vi "Actor Core.vi"(8 "error in":errorcluster, 11 "Test Actor in":refnum<class "Test Actor.lvclass">) -> (0 "error out":errorcluster, 3 "Actor out":refnum<class "Actor.lvclass">)   [LabVIEW 2020, in "Test.lvlib" / "Test Actor.lvclass"]
doc: "(<B>Filename</B>: Actor Framework.lvlib:Actor.lvclass:Actor Core.vi)\n\nReceives messages to the actor, reacts to them, and initiates any error handling that may shut the actor down.\n\nDescendant classes may override this VI to append parallel tasks for the actor to complete while it handles messages. Overrides use the Call Parent Method node."
uses:
  Test Actor.lvclass
  C:/Current projects/WS/PPL/HDH.Actor Framework.Core.Actor.lvlibp/1abvi3w/vi.lib/ActorFramework/Actor/Actor.lvclass
  PPL/HDH.Actor Framework.Core.Actor.lvlibp/1abvi3w/vi.lib/ActorFramework/Actor/Actor.lvclass
  PPL/HDH.Actor Framework.Core.Publisher.lvlibp/Messages/Response Msg/Response Core/Controls/Ctl_SendFunction.ctl
  PPL/HDH.Actor Framework.Core.Data Tracker.lvlibp/Messages for this Actor/Data Tracker Msg/Controls/Ctl_Action.ctl
  Test Actor.lvclass/Test Actor.ctl
  PPL/HDH.Actor Framework.Core.Graph.lvlibp/Graph/Graph.lvclass
  PPL/HDH.Actor Framework.Core.File Writer.lvlibp/File Writer/File Writer.lvclass
  PPL/HDH.Actor Framework.Core.File Writer.lvlibp/File Writer/File Post Action/File Post Action.lvclass
  Message/Test Instrument Msg/Test Instrument Msg.lvclass
  C:/Current projects/WS/PPL/HDH.Actor Framework.Core.Instrument Handler.lvlibp/Messages/Instrument Msg/Instrument Msg.lvclass
  Message/Test Multi Instrument Msg/Test Multi Instrument Msg.lvclass
  Message/Test Nested Multi Instrument Msg/Test Nested Multi Instrument Msg.lvclass
  PPL/HDH.Actor Framework.Core.Instrument Handler.lvlibp/Instrument Handler/Instrument Handler.lvclass
  PPL/HDH.Actor Framework.Core.Data Tracker.lvlibp/Data Tracker/Data Tracker.lvclass
  PPL/HDH.Actor Framework.Core.Actor.lvlibp/1abvi3w/vi.lib/ActorFramework/Message Enqueuer/Message Priority.ctl
  PPL/HDH.Actor Framework.Core.Data Tracker.lvlibp/Data Tracker/Data/Tracker Data.lvclass
  Message/Test Double Data Tracker/Test Double Data Tracker.lvclass
  C:/Current projects/WS/PPL/HDH.Actor Framework.Core.Publisher.lvlibp/Messages/Response Msg/Response Msg.lvclass
  Instrument/Test Instrument/Test Instrument.lvclass
  PPL/HDH.Actor Framework.Core.Instrument Driver.lvlibp/Instrument Driver/Controls/Ctl_ConnectionType.ctl
  Data/Test Double Data/Test Double Data.lvclass/Test Double Data.ctl
  Data/Test Double Data/Test Double Data.lvclass
  PPL/HDH.Actor Framework.Core.Msg.lvlibp/Sub Panel Insertion Msg/Sub Panel Insertion Msg.lvclass
  C:/Current projects/WS/PPL/HDH.Actor Framework.Core.Actor.lvlibp/1abvi3w/vi.lib/ActorFramework/Message/Message.lvclass
  PPL/HDH.Actor Framework.Core.File Writer.lvlibp/File Writer Messages/Open File Msg/Open File Msg.lvclass
  PPL/HDH.Actor Framework.Core.File Writer.lvlibp/File Writer Messages/Close File Msg/Close File Msg.lvclass
  PPL/HDH.Actor Framework.Core.Instrument Handler.lvlibp/Messages/Instrument Msg/Instrument Msg.lvclass
  PPL/HDH.Actor Framework.Core.Publisher.lvlibp/Publisher Messages/Targetted Msg/Targetted Msg.lvclass
  C:/Current projects/WS/PPL/HDH.Actor Framework.Core.Publisher.lvlibp/Publisher Messages/Sender Msg/Sender Msg.lvclass
  PPL/HDH.Actor Framework.Core.Instrument Handler.lvlibp/Instrument Handler Messages/Register Instrument Msg/Register Instrument Msg.lvclass
  PPL/HDH.Actor Framework.Core.Sequencer.lvlibp/Sequencer/Sequencer.lvclass
  PPL/HDH.Data.Generic.lvlibp/Data.lvclass
  PPL/HDH.Data.Generic.lvlibp/Generic Data/Generic Data.lvclass
  PPL/HDH.Actor Framework.Core.Actor.lvlibp/1abvi3w/vi.lib/ActorFramework/Stop Msg/Stop Msg.lvclass
  PPL/HDH.Actor Framework.Core.Sequencer.lvlibp
  PPL/HDH.Actor Framework.Core.Actor.lvlibp/1abvi3w/vi.lib/ActorFramework/Message Enqueuer/Message Enqueuer.lvclass
  PPL/HDH.Actor Framework.Core.Publisher.lvlibp/Publisher Messages/Publish Msg/Publish Msg.lvclass
  PPL/HDH.Actor Framework.Core.Instrument Driver.lvlibp/Instrument Driver/Instrument Driver.lvclass
  PPL/HDH.Actor Framework.Core.Publisher.lvlibp/Messages/Response Msg/Response Msg.lvclass
  PPL/HDH.Actor Framework.Core.Data Repository.lvlibp
  PPL/HDH.Actor Framework.Core.Data Tracker.lvlibp/Messages for this Actor/Data Tracker Msg/Data Tracker Msg.lvclass
  C:/Current projects/WS/PPL/HDH.Actor Framework.Core.Sequencer.lvlibp/Sequencer/Sequencer.lvclass
  C:/Current projects/WS/PPL/HDH.Actor Framework.Core.Data Tracker.lvlibp/Messages for this Actor/Data Tracker Msg/Data Tracker Msg.lvclass
  C:/Current projects/WS/PPL/HDH.Data.Generic.lvlibp/Data.lvclass
  PPL/HDH.Actor Framework.Core.Sequencer.lvlibp/Sequencer Messages/Batch Msg/Batch Msg.lvclass
  PPL/HDH.Actor Framework.Core.Publisher.lvlibp
  PPL/HDH.Actor Framework.Core.Data Tracker.lvlibp
panel:
  in  "Tab Control":T1(tab)
  in  "Send to tracker":bool
  in  "Send Function - Data Tracker":T2
  in  "Timeout if waiting(-1ms) - Data Tracker":i32=-1
  in  "Action(Start)":T3
  out "Data":string[](array[string])
  in  "Show data from repository":bool
  out "Success?":bool
  out "Found 'Test Double Data'":waveform(dbl)[](array[waveform])
  in  "Show data":bool
  in  "Stop Save":bool
  in  "Start Save":bool
  in  "File Path Control":path
  in  "Data":dbl[](array[numeric])
  in  "Publish Data to Graph":bool
  in  "Insert Graph":bool
  out "Recieved Data":waveform(dbl)[](graph)
  in  "Create Instrument":bool
  in  "Send Instrument Msg":bool
  in  "Publish Data?":bool=TRUE
  in  "Timeout if waiting(-1ms)":i32=-1
  in  "Send Function":T2
  in  "Msg Type":T4(ring)=enum."Test Nested Multi Instrument Msg"
  in  "Commit":bool
  in  "Setup Name":string
  in  "Single element?":bool
  in  "Tab Control 2":enum32{"String", "Double"}(tab)
  in  "String Array":string[](array[string])
  in  "Double Array":dbl[](array[numeric])
  out "replaced?":bool
  in  "Play Sequence":bool
  in  "Stop":bool
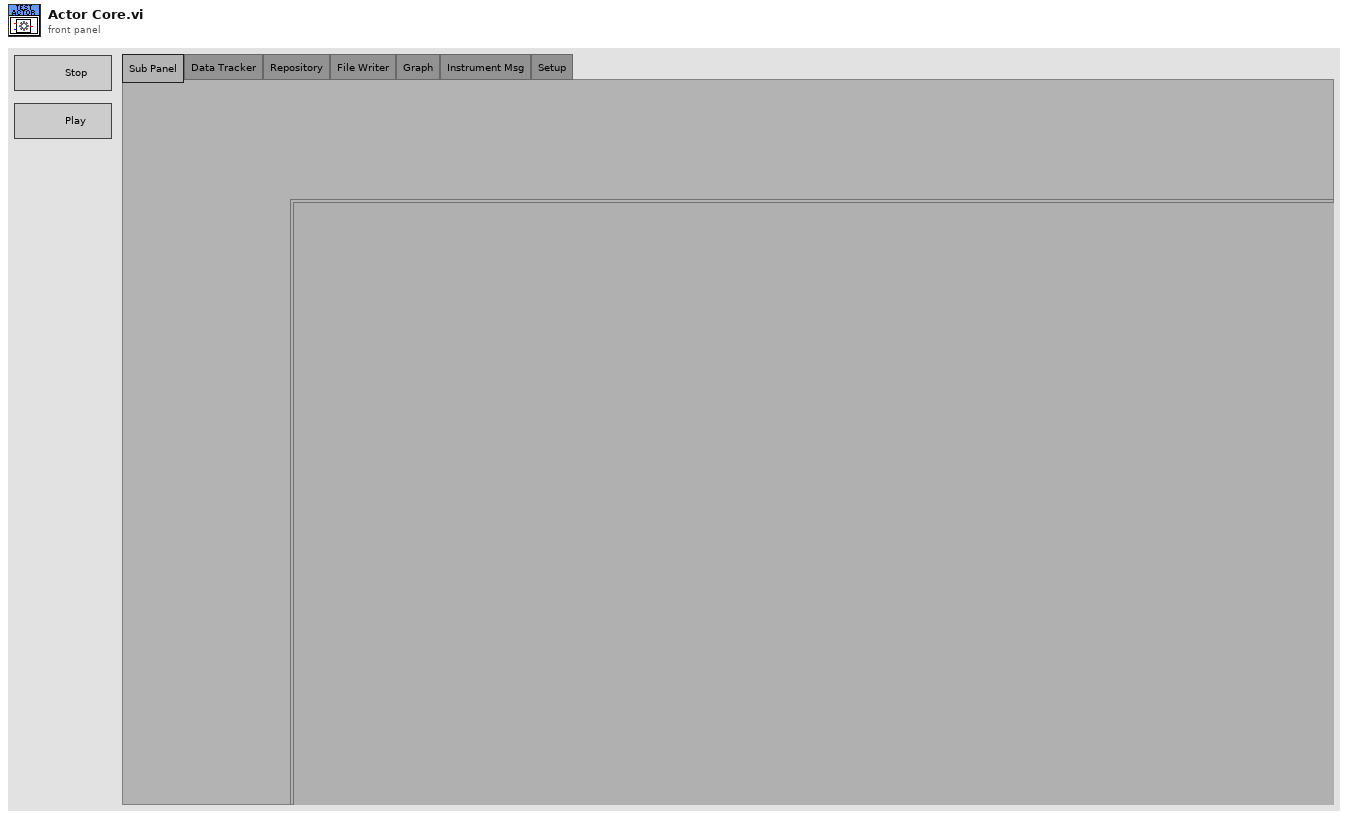
[diagram p1: front panel]
types:
  T1 = enum32{"Sub Panel", "Data Tracker", "Repository", "File Writer", "Graph", "Instrument Msg", "Setup"}
  T2 = typedef "HDH.Actor Framework.Core.Publisher.lvlibp/Ctl_SendFunction.ctl" = enum16{"Send and Forget", "Request Reply", "Await Reply"}
  T3 = typedef "HDH.Actor Framework.Core.Data Tracker.lvlibp/Ctl_Action.ctl" = enum16{"Start Tracking", "End Tracking", "Abort Tracking"}
  T4 = enum16{"Test Instrument Msg", "Test Multi Instrument Msg", "Test Nested Multi Instrument Msg"}
  T5 = enum32{"Invalid", "Standard", "Closed", "Hidden", "Minimized", "Maximized"}
  T6 = typedef "HDH.Actor Framework.Core.Instrument Driver.lvlibp/Instrument Driver.lvclass/Ctl_ConnectionType.ctl" = enum16{"BuiltIn/System", "PXI/PCI", "USB", "GPIB", "VXI", "Serial", "TCP/IP", "cRIO", "SCXI", "cDAQ", "SwitchBlock", "SCC", "FireWire", "Accessory", "CAN", "SwitchBlock Device"}
  T7 = typedef "HDH.Actor Framework.Core.Actor.lvlibp/Message Enqueuer.lvclass/Message Priority.ctl" = enum16{"Low", "Normal", "High"}
  T8 = typedef "HDH.Actor Framework.Core.Sequencer.lvlibp/Ctl_SequenceElement.ctl" = cluster{"Message Base Name":string, "Message Path":path, "Supports Data Access?":bool, "List Symbol":i32, "Sequence Control Element Array":T9[]}
  T9 = typedef "HDH.Actor Framework.Core.Sequencer.lvlibp/Ctl_SequenceControlElement.ctl" = cluster{"Data Override name":string, "Looped Override?":bool, "Control element":T10, "List Symbol":i32}
  T10 = typedef "HDH.Actor Framework.Core.Msg.lvlibp/Ctl_Control Element.ctl" = cluster{"Index":i32, "Label":string, "Value":variant}
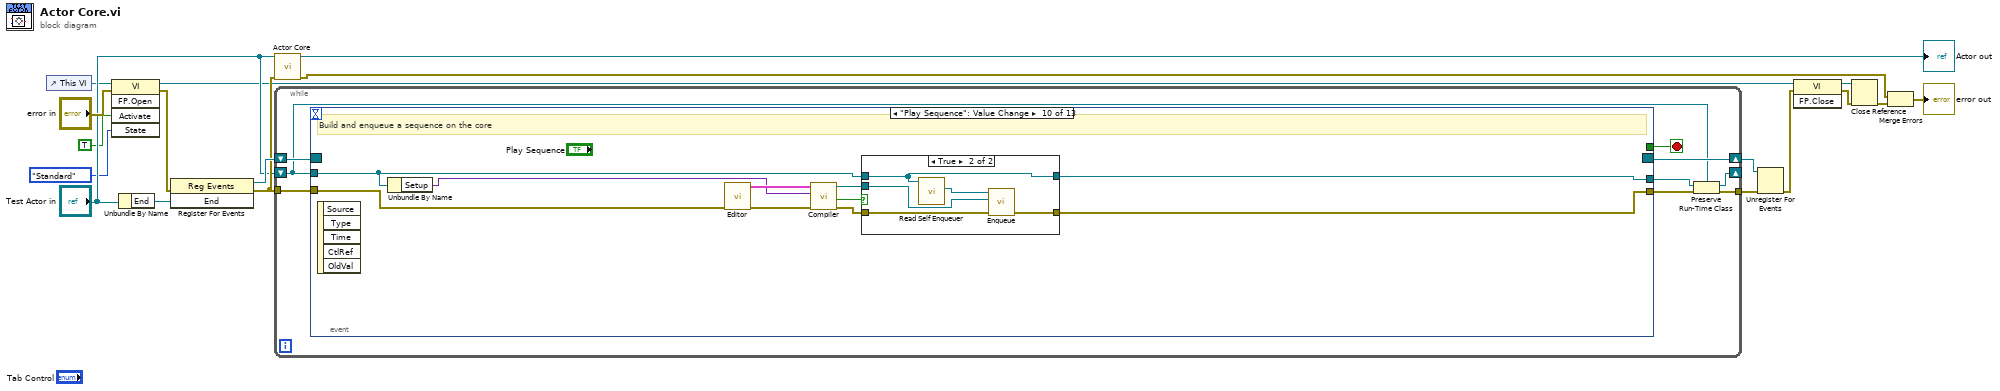
[diagram p0: block diagram]
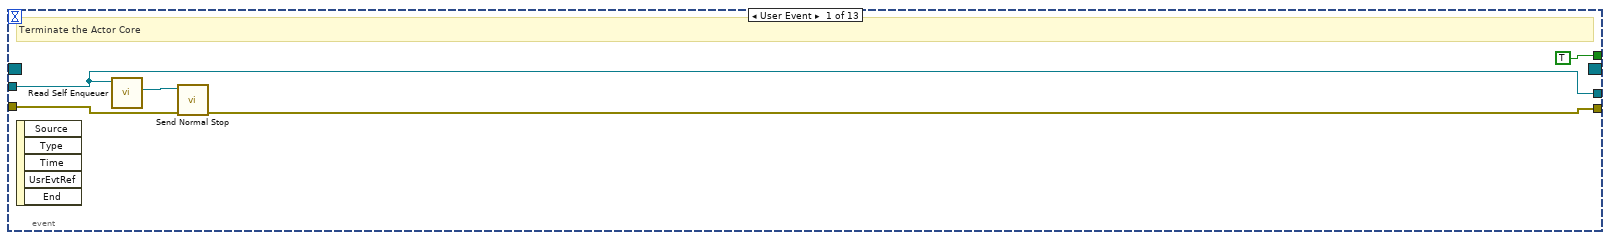
[diagram p2: hidden frame]
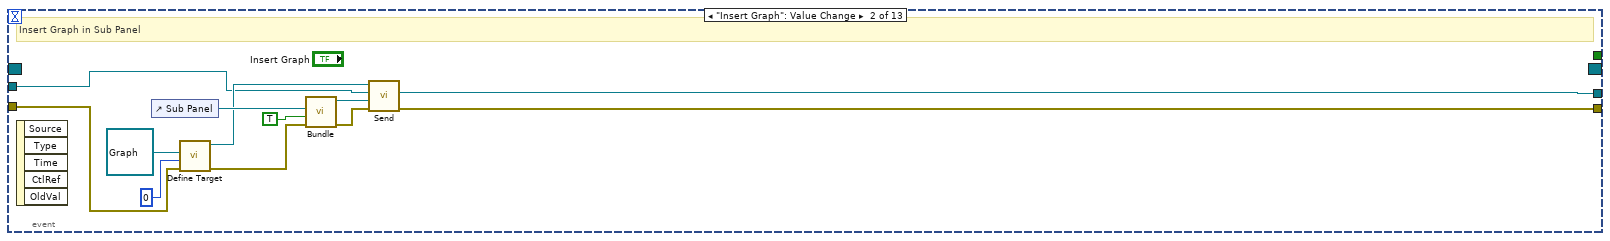
[diagram p3: hidden frame]
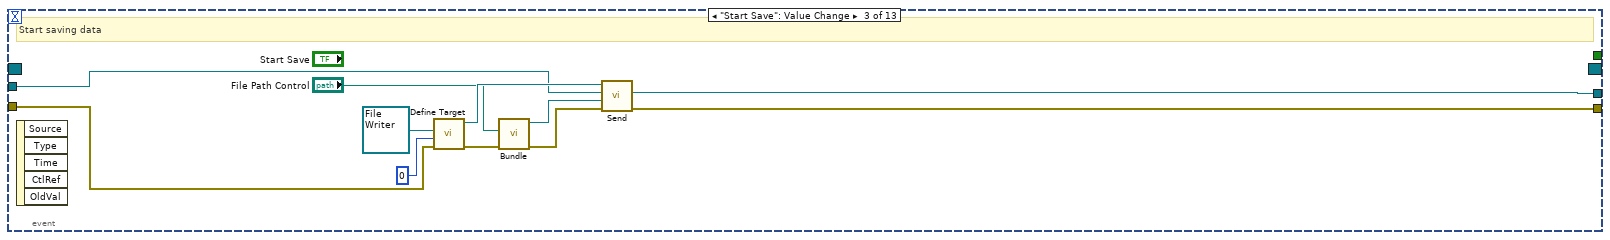
[diagram p4: hidden frame]
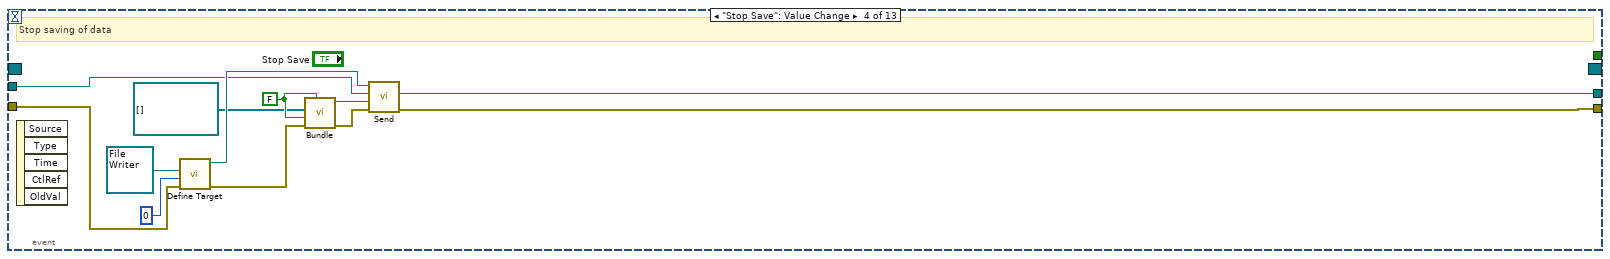
[diagram p5: hidden frame]
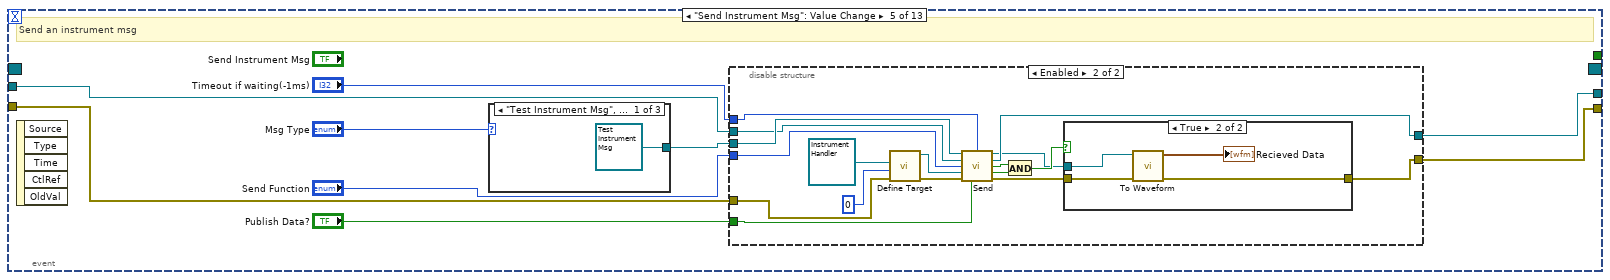
[diagram p6: hidden frame]
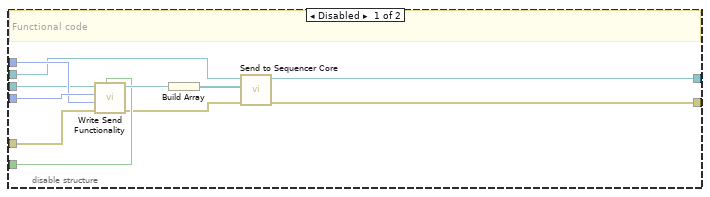
[diagram p7: hidden frame]
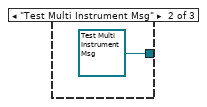
[diagram p9: hidden frame]
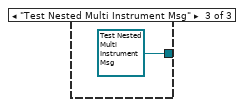
[diagram p10: hidden frame]
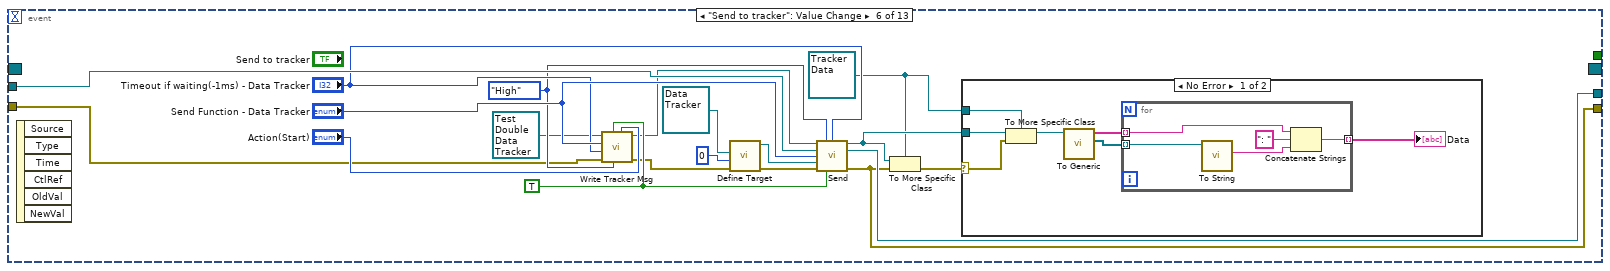
[diagram p11: hidden frame]
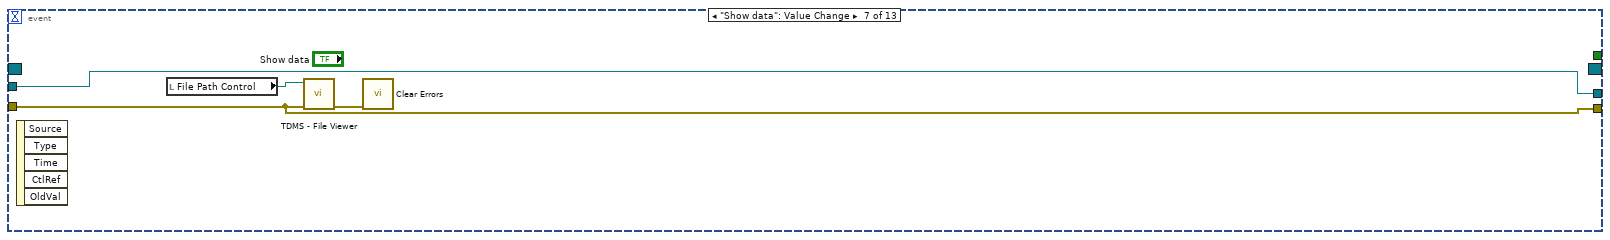
[diagram p13: hidden frame]
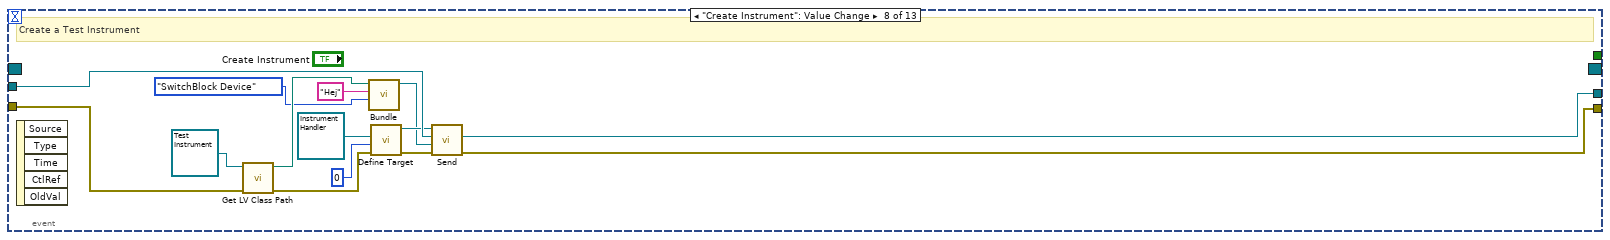
[diagram p14: hidden frame]
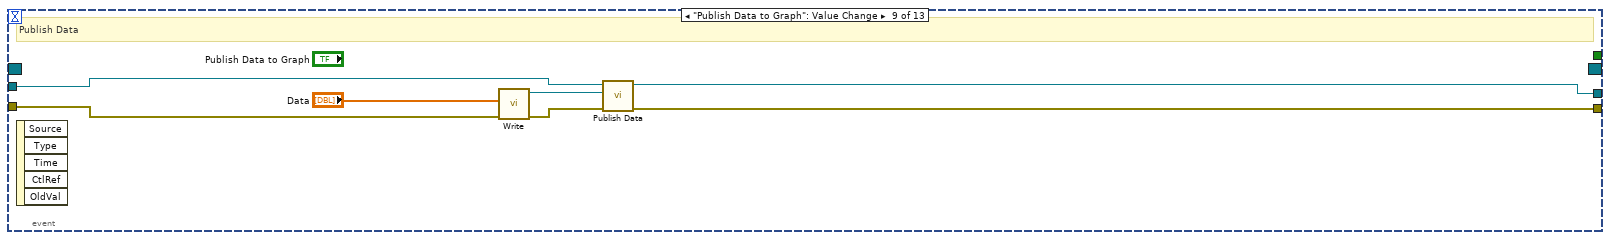
[diagram p15: hidden frame]
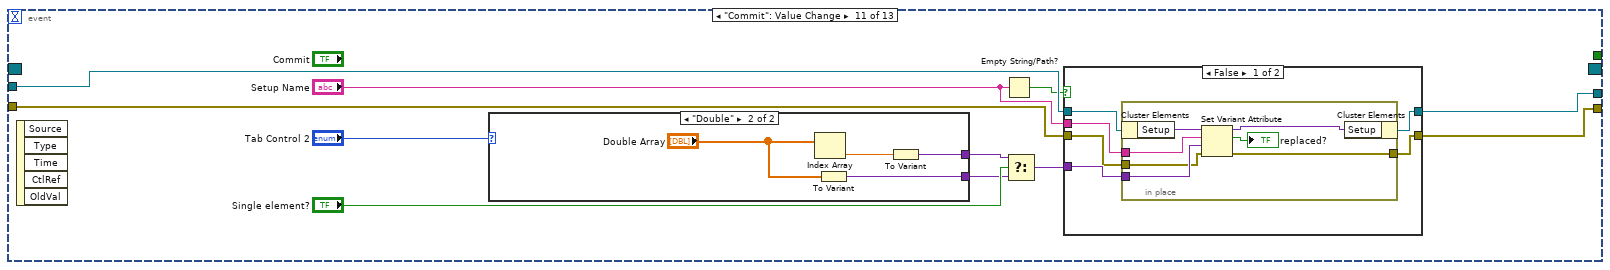
[diagram p17: hidden frame]
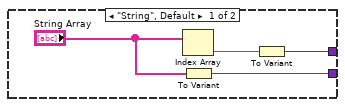
[diagram p19: hidden frame]
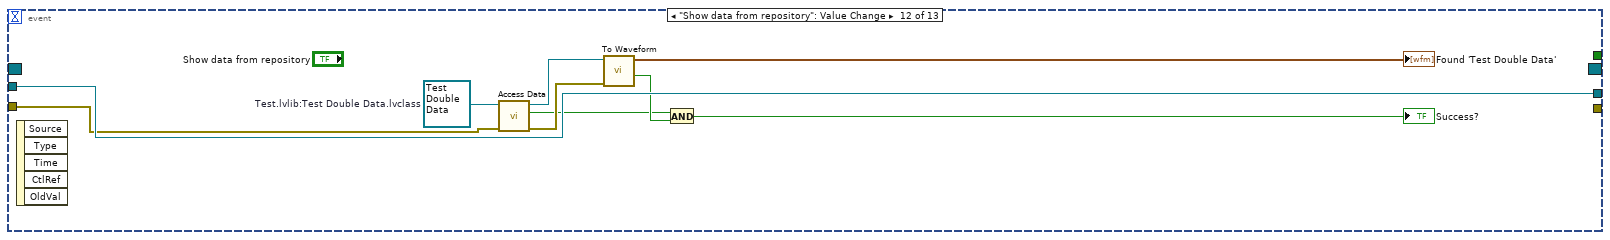
[diagram p20: hidden frame]
diagram:
  n1 = control-ref of="This VI"() -> (w8:refnum<vi>)
  n2 = invoke class="VI" method="FP.Open"(reference=w8, error in="error in", "Activate"=TRUE ("Activate?"), "State"=T5."Standard") -> (reference out=w3:refnum<vi>, error out=w9:errorcluster)  [unwired: 1 in, 3 out]
  n3 = Unbundle By Name("Test Actor in") -> ("End"=w18:refnum<user-event>)
  n4 = register-events(error in=w9, w18) -> (reference out=w16:refnum<event-registration>, error out=w12:errorcluster)  [unwired: 1 in]
  n5 = call-parent "Actor Core.vi"("error in"=w12, "Sequencer in"="Test Actor in") -> ("error out"=w14:errorcluster, "Actor out"=→"Actor out":refnum<class "Actor.lvclass">)  [unwired: 8 in]
  n6 = while {
    shift-right: [w27] -> w15
    shift-left: w16 -> [w28]
    shift-right: [w21] -> _
    shift-left: "Test Actor in" -> [w20]
    tunnel: w12 -> [w24]
    tunnel: [w23] -> w10
    stop <- w26 stop-if-true
    n7 = event shown="[9] \"Play Sequence\": Value Change" {
      selector: w28 -> [_ _ _ _ _ _ _ _ _ _ _ _ _]
      dyn-events: [_ _ _ _ _ _ _ _ _ _ _ _ _] -> w27
      timeout: _ -> [_ _ _ _ _ _ _ _ _ _ _ _ _]
      tunnel: [TRUE _ _ _ _ _ _ _ _ _ _ _ _] -> w26
      tunnel: w20 -> [w32 w36 w53 w65 w72 w128 w145 w155 w167 w171 w196 w229 w232]
      tunnel: [w32 w35 w52 w64 w71 w127 w145 w149 w166 w172 w187 w229 w232] -> w22
      tunnel: [w29 w34 w46 w58 w73 w118 w146 w150 w165 w175 w188 _ w230] -> w25
      tunnel: w24 -> [w30 w41 w51 w61 w77 w121 w146 w158 w164 w179 w189 w228 w231]
      event User Event {
        # "Terminate the Actor Core"
        n8 = event-data() -> ()  [unwired: 1 in, 5 out]
        n9 = call "Read Self Enqueuer.vi"("Actor"=w32) -> ("Self Enqueuer"=w31:refnum<class "Message Enqueuer.lvclass">)  [unwired: 10 in]
        n10 = call "Send Normal Stop.vi"("error in (no error)"=w30, "Message Enqueuer"=w31) -> ("error out"=w29:errorcluster)  [unwired: 9 in]
      }
      event "Insert Graph": Value Change {
        # "Insert Graph in Sub Panel"
        n11 = event-data() -> ()  [unwired: 1 in, 5 out]
        n12 = control-ref of="Sub Panel"() -> (w44:refnum<vi>)
        n13 = call "Define Target.vi"("error in (no error)"=w41, "Target Actor index(-1, all)"=0, "Target Actor"=refnum<class "Graph.lvclass"> refnum ("HDH.Actor Framework.Core.Graph.lvlibp:Graph.lvclass")) -> ("error out"=w40:errorcluster, "Targetted Msg out"=w38:refnum<class "Targetted Msg.lvclass">)  [unwired: 7 in]
        n14 = call "Bundle.vi"("error in (no error)"=w40, "Close reference after insertion(F)"=TRUE, "Sub Panel"=w44) -> ("error out"=w39:errorcluster, "Sub Panel Insertion Msg out"=w37:refnum<class "Sub Panel Insertion Msg.lvclass">)  [unwired: 7 in]
        n15 = call-dynamic "Send.vi"("error in (no error)"=w39, "Message"=w37, "Actor in"=w36, "Targetted Msg in"=w38) -> ("error out"=w34:errorcluster, "Actor out"=w35:refnum<class "Actor.lvclass">)  [unwired: 5 in, 1 out]
      }
      event "Start Save": Value Change {
        # "Start saving data"
        n16 = event-data() -> ()  [unwired: 1 in, 5 out]
        n17 = call "Define Target.vi"("error in (no error)"=w51, "Target Actor index(-1, all)"=0, "Target Actor"=refnum<class "File Writer.lvclass"> refnum ("HDH.Actor Framework.Core.File Writer.lvlibp:File Writer.lvclass")) -> ("error out"=w50:errorcluster, "Targetted Msg out"=w54:refnum<class "Targetted Msg.lvclass">)  [unwired: 7 in]
        n18 = call "Bundle.vi"("error in (no error)"=w50, "New File Path"="File Path Control") -> ("error out"=w48:errorcluster, "Open File Msg out"=w47:refnum<class "Open File Msg.lvclass">)  [unwired: 8 in]
        n19 = call-dynamic "Send.vi"("error in (no error)"=w48, "Message"=w47, "Actor in"=w53, "Targetted Msg in"=w54) -> ("error out"=w46:errorcluster, "Actor out"=w52:refnum<class "Actor.lvclass">)  [unwired: 5 in, 1 out]
      }
      event "Stop Save": Value Change {
        w63 = FALSE ("Perform Post Actions?(T)")
        # "Stop saving of data"
        n20 = event-data() -> ()  [unwired: 1 in, 5 out]
        n21 = call "Define Target.vi"("error in (no error)"=w61, "Target Actor index(-1, all)"=0, "Target Actor"=refnum<class "File Writer.lvclass"> refnum ("HDH.Actor Framework.Core.File Writer.lvlibp:File Writer.lvclass")) -> ("error out"=w60:errorcluster, "Targetted Msg out"=w66:refnum<class "Targetted Msg.lvclass">)  [unwired: 7 in]
        n22 = call "Bundle.vi"("Await Completion?(F)"=w63, "error in (no error)"=w60, "Perform Post Actions?(T)"=w63, "File Post Action"=refnum<class "File Post Action.lvclass">[] []) -> ("error out"=w59:errorcluster, "Close File Msg out"=w62:refnum<class "Close File Msg.lvclass">)  [unwired: 6 in]
        n23 = call-dynamic "Send.vi"("error in (no error)"=w59, "Message"=w62, "Actor in"=w65, "Targetted Msg in"=w66) -> ("error out"=w58:errorcluster, "Actor out"=w64:refnum<class "Actor.lvclass">)  [unwired: 5 in, 1 out]
      }
      event "Send Instrument Msg": Value Change {
        # "Send an instrument msg"
        n24 = event-data() -> ()  [unwired: 1 in, 5 out]
        n25 = case shown="\"Test Instrument Msg\", Default" "Msg Type" {
          tunnel: [refnum<class "Test Instrument Msg.lvclass"> refnum ("Test.lvlib:Test Instrument Msg.lvclass") refnum<class "Test Multi Instrument Msg.lvclass"> refnum ("Test.lvlib:Test Multi Instrument Msg.lvclass") refnum<class "Test Nested Multi Instrument Msg.lvclass"> refnum ("Test.lvlib:Test Nested Multi Instrument Msg.lvclass")] -> w69
          frame "Test Instrument Msg", Default {
          }
          frame "Test Multi Instrument Msg" {
          }
          frame "Test Nested Multi Instrument Msg" {
          }
        }
        n26 = disable-structure shown="Enabled" {
          disable-tunnel: w77 -> [w88 w97]
          disable-tunnel: "Send Function" -> [w85 w103]
          disable-tunnel: "Timeout if waiting(-1ms)" -> [w84 w104]
          disable-tunnel: "Publish Data?" -> [w83 w102]
          disable-tunnel: [w81 w89] -> w73
          disable-tunnel: w72 -> [w80 w101]
          disable-tunnel: [w79 w100] -> w71
          disable-tunnel: w69 -> [w78 w105]
          frame Disabled {
            # "Functional code"
            n27 = call "Write Send Functionality.vi"("Publish Data?(T)"=w83, "error in (no error)"=w88, "Timeout if Waiting(-1ms)"=w84, "Send Function(Await Reply)"=w85, "Instrument Msg in"=w78) -> ("error out"=w82:errorcluster, "Instrument Msg out"=w87:refnum<class "Instrument Msg.lvclass">)  [unwired: 5 in]
            n28 = Build Array(w87) -> (w86:refnum<class "Instrument Msg.lvclass">[])
            n29 = call "Send to Sequencer Core.vi"("error in (no error)"=w82, "Message Array"=w86, "Sequencer in"=w80) -> ("error out"=w81:errorcluster, "Sequencer out"=w79:refnum<class "Test Actor.lvclass">)  [unwired: 7 in]
          }
          frame Enabled {
            n30 = call "Define Target.vi"("error in (no error)"=w97, "Target Actor index(-1, all)"=0, "Target Actor"=refnum<class "Instrument Handler.lvclass"> refnum ("HDH.Actor Framework.Core.Instrument Handler.lvlibp:Instrument Handler.lvclass")) -> ("error out"=w96:errorcluster, "Targetted Msg out"=w98:refnum<class "Targetted Msg.lvclass">)  [unwired: 7 in]
            n31 = call "Send.vi"("Response Msg in"=w105, "Timeout if waiting(-1ms)"=w104, "Actor in"=w101, "Send Function"=w103, "Sender (publish)"=w98, "error in (no error)"=w96, "Publish Data?(F)"=w102) -> ("Data"=w91:refnum<class "Data.lvclass">, "Actor out"=w100:refnum<class "Actor.lvclass">, "Success?"=w94:bool, "Waited?"=w93:bool, "error out"=w90:errorcluster)  [unwired: 4 in]
            n32 = And(x=w94, y=w93) -> (x .and. y?=w92:bool)
            n33 = case shown="True" w92 {
              tunnel: w91 -> [_ w110]
              tunnel: w90 -> [w106 w108]
              tunnel: [w106 w107] -> w89
              frame False {
              }
              frame True {
                n34 = call-dynamic "To Waveform.vi"("error in (no error)"=w108, "Data in"=w110) -> ("error out"=w107:errorcluster, "Waveform Array"=→"Recieved Data":waveform(dbl)[])  [unwired: 7 in, 1 out]
              }
            }
          }
        }
      }
      event "Send to tracker": Value Change {
        w115 = refnum<class "Tracker Data.lvclass"> refnum ("HDH.Actor Framework.Core.Data Tracker.lvlibp:Tracker Data.lvclass")
        w126 = TRUE ("Publish Data?(F)")
        w122 = Message_Priority."High" ("Message Priority (Normal)")
        n35 = event-data() -> ()  [unwired: 1 in, 6 out]
        n36 = call "Write Tracker Msg.vi"("Action(Start)"="Action(Start)", "Message Priority(Normal)"=w122, "Publish Data?(T)"=w126, "error in (no error)"=w121, "Timeout if Waiting(-1ms)"="Timeout if waiting(-1ms) - Data Tracker", "Send Function(Await Reply)"="Send Function - Data Tracker", "Data Tracker Msg in"=refnum<class "Test Double Data Tracker.lvclass"> refnum ("Test.lvlib:Test Double Data Tracker.lvclass")) -> ("error out"=w120:errorcluster, "Data Tracker Msg out"=w119:refnum<class "Test Double Data Tracker.lvclass">)  [unwired: 3 in]
        n37 = call "Define Target.vi"("error in (no error)"=w120, "Target Actor index(-1, all)"=0, "Target Actor"=refnum<class "Data Tracker.lvclass"> refnum ("HDH.Actor Framework.Core.Data Tracker.lvlibp:Data Tracker.lvclass")) -> ("error out"=w129:errorcluster, "Targetted Msg out"=w132:refnum<class "Targetted Msg.lvclass">)  [unwired: 7 in]
        n38 = call "Send.vi"("Response Msg in"=w119, "Message Priority (Normal)"=w122, "Timeout if waiting(-1ms)"="Timeout if waiting(-1ms) - Data Tracker", "Actor in"=w128, "Send Function"="Send Function - Data Tracker", "Sender (publish)"=w132, "error in (no error)"=w129, "Publish Data?(F)"=w126) -> ("Data"=w116:refnum<class "Data.lvclass">, "Actor out"=w127:refnum<class "Actor.lvclass">, "error out"=w118:errorcluster)  [unwired: 3 in, 2 out]
        n39 = To More Specific Class(target class=w115, reference=w116, error in=w118) -> (error out=w117:errorcluster)  [unwired: 1 out]
        n40 = case shown="No Error" w117 {
          selector: w117 -> [w139 _]
          tunnel: w116 -> [w138 _]
          tunnel: w115 -> [w137 _]
          frame No Error {
            n41 = To More Specific Class(target class=w137, reference=w138, error in=w139) -> (specific class reference=w136:refnum<class "Tracker Data.lvclass">)  [unwired: 1 out]
            n42 = call-dynamic "To Generic.vi"("Request Data in"=w136) -> ("Generic Data"=w135:refnum<class "Generic Data.lvclass">[], "Data Name"=w134:string[])  [unwired: 8 in, 1 out]
            n43 = for {
              tunnel: w135 -> [w144] mode=indexing
              tunnel: w134 -> [w143] mode=indexing
              tunnel: [w140] -> w133 mode=indexing
              n44 = call-dynamic "To String.vi"("Generic Data in"=w144) -> ("String"=w141:string)  [unwired: 9 in, 1 out]
              n45 = Concatenate Strings(w143, ": " ("string"), w141) -> (w140:string)
            }
            "Data" <- w133
          }
          frame Error {
          }
        }
      }
      event "Show data": Value Change {
        n46 = event-data() -> ()  [unwired: 1 in, 5 out]
        n47 = local read "File Path Control"() -> (w148:path)
        n48 = call <vilib>:"TDMS - File Viewer.vi"("error in (no error)"=w146, "file path"=w148) -> ("error out"=w147:errorcluster)  [unwired: 4 in, 1 out]
        n49 = call <vilib>:"Clear Errors.vi"("error in (no error)"=w147) -> ()  [unwired: 5 in, 2 out]
      }
      event "Create Instrument": Value Change {
        # "Create a Test Instrument"
        n50 = event-data() -> ()  [unwired: 1 in, 5 out]
        n51 = call <vilib>:"Get LV Class Path.vi"("error in (no error)"=w158, "object"=refnum<class "Test Instrument.lvclass"> refnum ("Test.lvlib:Test Instrument.lvclass")) -> ("error out"=w152:errorcluster, "class path"=w160:path)  [unwired: 8 in]
        n52 = call "Bundle.vi"("Connection Type"=Ctl_ConnectionType."SwitchBlock Device", "Alias"="Hej", "Driver Path"=w160) -> ("Register Instrument Msg out"=w153:refnum<class "Register Instrument Msg.lvclass">)  [unwired: 8 in]
        n53 = call "Define Target.vi"("error in (no error)"=w152, "Target Actor index(-1, all)"=0, "Target Actor"=refnum<class "Instrument Handler.lvclass"> refnum ("HDH.Actor Framework.Core.Instrument Handler.lvlibp:Instrument Handler.lvclass")) -> ("error out"=w151:errorcluster, "Targetted Msg out"=w154:refnum<class "Targetted Msg.lvclass">)  [unwired: 7 in]
        n54 = call-dynamic "Send.vi"("error in (no error)"=w151, "Message"=w153, "Actor in"=w155, "Targetted Msg in"=w154) -> ("error out"=w150:errorcluster, "Actor out"=w149:refnum<class "Actor.lvclass">)  [unwired: 5 in, 1 out]
      }
      event "Publish Data to Graph": Value Change {
        # "Publish Data"
        n55 = event-data() -> ()  [unwired: 1 in, 5 out]
        n56 = call "Write.vi"("error in (no error)"=w164, "Data"="Data") -> ("error out"=w163:errorcluster, "Test Double Data out"=w168:refnum<class "Test Double Data.lvclass">)  [unwired: 8 in]
        n57 = call "Publish Data.vi"("error in (no error)"=w163, "Data to Publish"=w168, "Actor in"=w167) -> ("error out"=w165:errorcluster, "Actor out"=w166:refnum<class "Test Actor.lvclass">)  [unwired: 6 in, 1 out]
      }
      event "Play Sequence": Value Change {
        # "Build and enqueue a sequence on the core"
        n58 = event-data() -> ()  [unwired: 1 in, 5 out]
        n59 = Unbundle By Name(w171) -> ("Setup"=w170:variant)
        n60 = call "Editor.vi"("error in (no error)"=w179) -> ("error out"=w177:errorcluster, "Uncompiled sequence out"=w178:T8[])  [unwired: 9 in]
        n61 = call "Compiler.vi"("error in (no error)"=w177, "Override Look up table"=w170, "Uncompiled sequence in"=w178) -> ("error out"=w174:errorcluster, "Success?"=w176:bool, "Batch Msg out"=w173:refnum<class "Batch Msg.lvclass">)  [unwired: 6 in]
        n62 = case shown="True" w176 {
          tunnel: [w181 w182] -> w175
          tunnel: w174 -> [w181 w183]
          tunnel: w173 -> [_ w184]
          tunnel: [w180 w186] -> w172
          tunnel: w171 -> [w180 w186]
          frame False {
          }
          frame True {
            n63 = call "Read Self Enqueuer.vi"("Actor"=w186) -> ("Self Enqueuer"=w185:refnum<class "Message Enqueuer.lvclass">)  [unwired: 10 in]
            n64 = call "Enqueue.vi"("error in (no error)"=w183, "Message"=w184, "Message Enqueuer in"=w185) -> ("error out"=w182:errorcluster)  [unwired: 7 in, 1 out]
          }
        }
      }
      event "Commit": Value Change {
        n65 = event-data() -> ()  [unwired: 1 in, 5 out]
        n66 = case shown="\"Double\"" "Tab Control 2" {
          tunnel: [w214 w219] -> w191
          tunnel: [w213 w217] -> w192
          frame "String", Default {
            n67 = Index Array(array="String Array") -> (element=w216:string)  [unwired: 1 in]
            n68 = To Variant(anything="String Array") -> (Variant=w214:variant)
            n69 = To Variant(anything=w216) -> (Variant=w213:variant)
          }
          frame "Double" {
            n70 = Index Array(array="Double Array") -> (element=w218:dbl)  [unwired: 1 in]
            n71 = To Variant(anything="Double Array") -> (Variant=w219:variant)
            n72 = To Variant(anything=w218) -> (Variant=w217:variant)
          }
        }
        n73 = Empty String/Path?(string/path="Setup Name") -> (empty?=w195:bool)
        n74 = Select(t=w192, s="Single element?", f=w191) -> (s? t:f=w190:variant)
        n75 = case shown="False" w195 {
          tunnel: w196 -> [w203 w211]
          tunnel: "Setup Name" -> [w202 _]
          tunnel: w190 -> [w201 _]
          tunnel: w189 -> [w200 w212]
          tunnel: [w199 w212] -> w188
          tunnel: [w198 w211] -> w187
          frame False {
            n76 = in-place {
              in-place-border: w202 -> [w208]
              in-place-border: w201 -> [w207]
              in-place-border: w200 -> [w206]
              in-place-border: [w205] -> w199
              n77 = in-place-cluster #1(w203) -> ("Setup"=w210:variant)
              n78 = Set Variant Attribute(Variant=w210, name=w208, value=w207, error in=w206) -> (Variant out=w209:variant, replaced=→"replaced?":bool, error out=w205:errorcluster)
              n79 = in-place-cluster #1("Setup"=w209) -> (w198:refnum<class "Test Actor.lvclass">)
            }
          }
          frame True {
          }
        }
      }
      event "Show data from repository": Value Change {
        w227 = refnum<class "Test Double Data.lvclass"> refnum  # Test.lvlib:Test Double Data.lvclass
        n80 = event-data() -> ()  [unwired: 1 in, 5 out]
        n81 = call "Access Data.vi"("error in (no error)"=w228, "Data to Access"=w227) -> ("error out"=w225:errorcluster, "Found?"=w222:bool, "Data out"=w226:refnum<class "Test Double Data.lvclass">)  [unwired: 7 in]
        n82 = call-dynamic "To Waveform.vi"("error in (no error)"=w225, "Test Double Data in"=w226) -> ("Success?"=w224:bool, "Waveform Array"=→"Found 'Test Double Data'":waveform(dbl)[])  [unwired: 7 in, 1 out]
        n83 = And(x=w222, y=w224) -> (x .and. y?=→"Success?":bool)
      }
      event "Stop": Value Change {
        # "Terminate the Application"
        n84 = event-data() -> ()  [unwired: 1 in, 5 out]
        n85 = call "Read Caller Enqueuer.vi"("Actor"=w232) -> ("Caller Enqueuer"=w233:refnum<class "Message Enqueuer.lvclass">)  [unwired: 10 in]
        n86 = call "Send Normal Stop.vi"("error in (no error)"=w231, "Message Enqueuer"=w233) -> ("error out"=w230:errorcluster)  [unwired: 9 in]
      }
    }
    n87 = Preserve Run-Time Class(object in=w22, error in=w25, 2:w20) -> (object out=w21:refnum<class "Test Actor.lvclass">, error out=w23:errorcluster)
  }
  n88 = Unregister For Events(event registration refnum=w15, error in=w10) -> (error out=w5:errorcluster)
  n89 = invoke class="VI" method="FP.Close"(reference=w3, error in=w5) -> (reference out=w1:refnum<vi>, error out=w4:errorcluster)  [unwired: 1 in, 1 out]
  n90 = Close Reference(reference=w1, error in (no error)=w4) -> (error out=w2:errorcluster)
  n91 = Merge Errors(w14, w2) -> (→"error out":errorcluster)
